vi "LinearFit.vi"(10 "index":i32[](array[numeric]), 11 "9dots":dbl[][](array[numeric])) -> (3 "slope":dbl caption="斜率" format="%#.6g")   [LabVIEW 2011]
uses:
  <vilib>/Analysis/NI_AALPro.lvlib
panel:
  out "9dots 2":dbl[][](array[numeric])
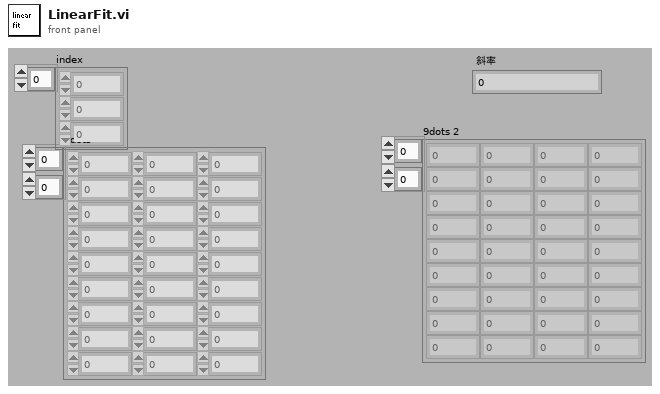
[diagram p1: front panel]
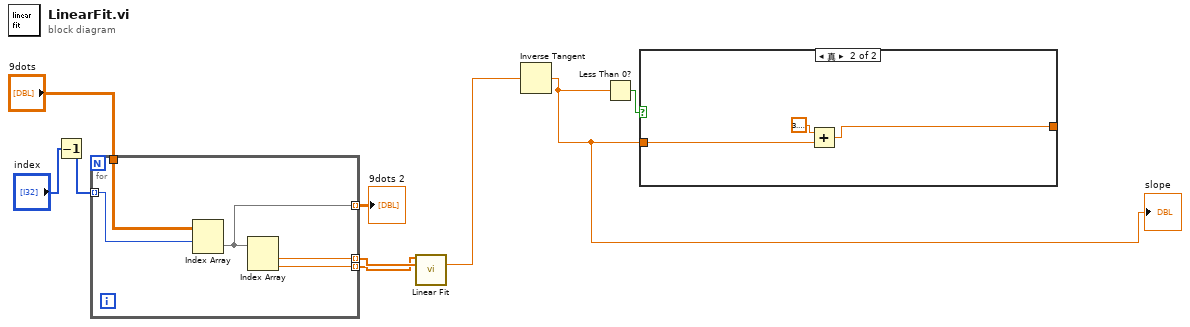
[diagram p0: block diagram]
diagram:
  n1 = Decrement(x="index") -> (x-1=w5:i32[])
  n2 = for {
    tunnel: w5 -> [w13] mode=indexing
    tunnel: "9dots" -> [w14]
    tunnel: [w12] -> w8 mode=indexing
    tunnel: [w11] -> w7 mode=indexing
    tunnel: [w10] -> w4 mode=indexing
    n3 = Index Array(array=w14, index (row)=w13) -> (element=w10:dbl[])  [unwired: 1 in]
    n4 = Index Array(array=w10) -> (element #1=w12:dbl, element #2=w11:dbl)  [unwired: 2 in]
  }
  "9dots 2" <- w4
  n5 = call <vilib>:"Linear Fit.vi"("Y"=w7, "X"=w8) -> ("slope"=w3:dbl)  [unwired: 4 in, 9 out]
  n6 = Inverse Tangent(1:w3) -> (0:w1:dbl)
  "slope" <- w1
  n7 = Less Than 0?(x=w1) -> (x < 0?=w2:bool)
  n8 = case shown="真" w2 {
    tunnel: w1 -> [w15 w17]
    tunnel: [w15 w16] -> _
    frame False {
    }
    frame True {
      n9 = Add(x=3.141592653589793, y=w17) -> (x+y=w16:dbl)
    }
  }
